vi "GlobalVariableData.vi"() -> ()   [LabVIEW 2023, in "LTT_TeststandSteptypes.lvlib"]
uses:
  LTT_TeststandSteptypes.lvlib
  PowerMonitor/Control/PowerData.ctl
panel:
  in  "Teststand Terminate?":bool
  out "Engine Enable":cluster{"Chamber Engine?":bool}
  in  "Chamber Temperature":T1
  out "PowerStatus":T2
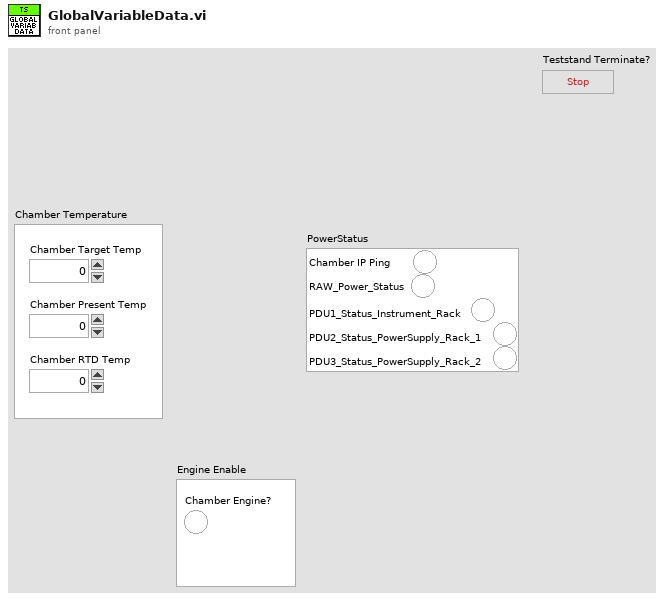
[diagram p1: front panel]
types:
  T1 = cluster{"Chamber Present Temp":dbl, "Chamber Target Temp":dbl, "Chamber RTD Temp":dbl}
  T2 = typedef "LTT_TeststandSteptypes.lvlib/PowerData.ctl" = cluster{"Chamber IP Ping":bool, "RAW_Power_Status":bool, "PDU1_Status_Instrument_Rack":bool, "PDU2_Status_PowerSupply_Rack_1":bool, "PDU3_Status_PowerSupply_Rack_2":bool}
diagram:
